vi "Listen.vi"(8 "error in (no error)":errorcluster, 10 "timeout in ms (-1)":i32=-1, 11 "event_input in":refnum<class "Event Input.lvclass">) -> (0 "error out":errorcluster, 1 "timed out?":bool, 2 "result":refnum<class "result.lvclass">, 3 "event_input out":refnum<class "Event Input.lvclass">)   [LabVIEW 2015, in "Event Input.lvclass"]
uses:
  Event Input.lvclass
  Result/result.lvclass
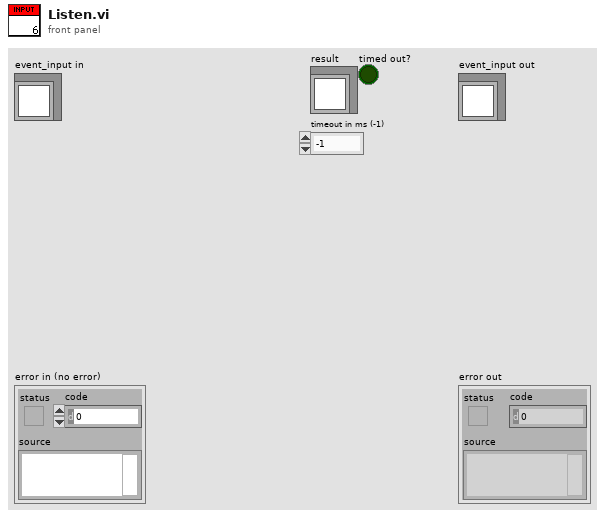
[diagram p1: front panel]
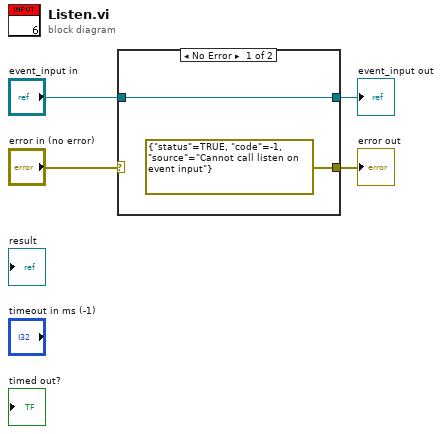
[diagram p0: block diagram]
diagram:
  n1 = case shown="No Error" "error in (no error)" {
    selector: "error in (no error)" -> [_ w7]
    tunnel: [w6 w8] -> w3
    tunnel: "event_input in" -> [w6 w8]
    tunnel: [errorcluster {"status"=TRUE, "code"=-1, "source"="Cannot call listen on event input"} ("error IO") w7] -> w1
    frame No Error {
    }
    frame Error {
    }
  }
  "error out" <- w1
  "event_input out" <- w3
